vi "DeviceConfigType_to_Byte.vi"(4 "DeviceConfig":T1) -> (1 "Byte Array":u8[](array[numeric]))   [LabVIEW 2020]
uses:
  <instrlib>/Devices/Avantes/clusterdef.ctl
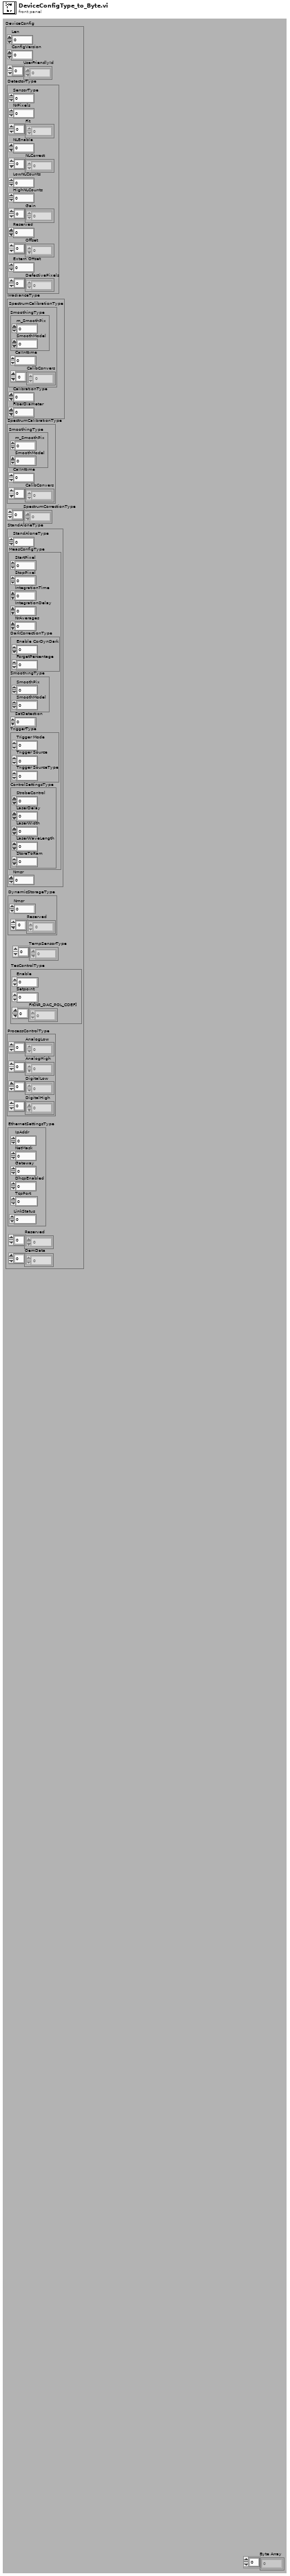
[diagram p1: front panel]
types:
  T1 = typedef "clusterdef.ctl" = cluster{"Len":u16, "ConfigVersion":u16, "UserFriendlyId":u8[], "DetectorType":cluster{"SensorType":u8, "NrPixels":u16, "Fit":sgl[], "NLEnable":u8, "NLCorrect":dbl[], "LowNLCounts":dbl, "HighNLCounts":dbl, "Gain":sgl[], "Reserved":sgl, "Offset":sgl[], "Extern Offset":sgl, "DefectivePixels":u16[]}, "IrradianceType":cluster{"SpectrumCalibrationType":cluster{"SmoothingType":cluster{"m_SmoothPix":u16, "SmoothModel":u8}, "CalInttime":sgl, "CalibConvers":sgl[]}, "CalibrationType":u8, "FiberDiameter":i32}, "SpectrumCalibrationType":cluster{"SmoothingType":cluster{"m_SmoothPix":u16, "SmoothModel":u8}, "CalInttime":sgl, "CalibConvers":sgl[]}, "SpectrumCorrectionType":sgl[], "StandAloneType":cluster{"StandAloneType":u8, "MeasConfigType":cluster{"StartPixel":u16, "StopPixel":u16, "IntegrationTime":sgl, "IntegrationDelay":u32, "NrAverages":u32, "DarkCorrectionType":cluster{"Enable CorDynDark":u8, "ForgetPercentage":u8}, "SmoothingType":cluster{"SmoothPix":u16, "SmoothModel":u8}, "SatDetection":u8, "TriggerType":cluster{"Trigger Mode":u8, "Trigger Source":u8, "Trigger SourceType":u8}, "ControlSettingsType":cluster{"StrobeControl":u16, "LaserDelay":u32, "LaserWidth":u32, "LaserWaveLength":sgl, "StoreToRam":u16}}, "Nmsr":i16}, "DynamicStorageType":cluster{"Nmsr":i32, "Reserved":u8[]}, "TempSensorType":sgl[], "TecControlType":cluster{"Enable":u8, "Setpoint":sgl, "Fit[NR_DAC_POL_COEF]":sgl[]}, "ProcessControlType":cluster{"AnalogLow":sgl[], "AnalogHigh":sgl[], "DigitalLow":sgl[], "DigitalHigh":sgl[]}, "EthernetSettingsType":cluster{"IpAddr":u32, "NetMask":u32, "Gateway":u32, "DhcpEnabled":u8, "TcpPort":u16, "LinkStatus":u8}, "Reserved":u8[], "OemData":u8[]}
  T2 = cluster{"SensorType":u8, "NrPixels":u16, "Fit":sgl[], "NLEnable":u8, "NLCorrect":dbl[], "LowNLCounts":dbl, "HighNLCounts":dbl, "Gain":sgl[], "Reserved":sgl, "Offset":sgl[], "Extern Offset":sgl, "DefectivePixels":u16[]}
  T3 = cluster{"SpectrumCalibrationType":cluster{"SmoothingType":cluster{"m_SmoothPix":u16, "SmoothModel":u8}, "CalInttime":sgl, "CalibConvers":sgl[]}, "CalibrationType":u8, "FiberDiameter":i32}
  T4 = cluster{"SmoothingType":cluster{"m_SmoothPix":u16, "SmoothModel":u8}, "CalInttime":sgl, "CalibConvers":sgl[]}
  T5 = cluster{"StandAloneType":u8, "MeasConfigType":cluster{"StartPixel":u16, "StopPixel":u16, "IntegrationTime":sgl, "IntegrationDelay":u32, "NrAverages":u32, "DarkCorrectionType":cluster{"Enable CorDynDark":u8, "ForgetPercentage":u8}, "SmoothingType":cluster{"SmoothPix":u16, "SmoothModel":u8}, "SatDetection":u8, "TriggerType":cluster{"Trigger Mode":u8, "Trigger Source":u8, "Trigger SourceType":u8}, "ControlSettingsType":cluster{"StrobeControl":u16, "LaserDelay":u32, "LaserWidth":u32, "LaserWaveLength":sgl, "StoreToRam":u16}}, "Nmsr":i16}
  T6 = cluster{"Enable":u8, "Setpoint":sgl, "Fit[NR_DAC_POL_COEF]":sgl[]}
  T7 = cluster{"AnalogLow":sgl[], "AnalogHigh":sgl[], "DigitalLow":sgl[], "DigitalHigh":sgl[]}
  T8 = cluster{"IpAddr":u32, "NetMask":u32, "Gateway":u32, "DhcpEnabled":u8, "TcpPort":u16, "LinkStatus":u8}
  T9 = cluster{"StartPixel":u16, "StopPixel":u16, "IntegrationTime":sgl, "IntegrationDelay":u32, "NrAverages":u32, "DarkCorrectionType":cluster{"Enable CorDynDark":u8, "ForgetPercentage":u8}, "SmoothingType":cluster{"SmoothPix":u16, "SmoothModel":u8}, "SatDetection":u8, "TriggerType":cluster{"Trigger Mode":u8, "Trigger Source":u8, "Trigger SourceType":u8}, "ControlSettingsType":cluster{"StrobeControl":u16, "LaserDelay":u32, "LaserWidth":u32, "LaserWaveLength":sgl, "StoreToRam":u16}}
  T10 = cluster{"Enable CorDynDark":u8, "ForgetPercentage":u8}
  T11 = cluster{"Trigger Mode":u8, "Trigger Source":u8, "Trigger SourceType":u8}
  T12 = cluster{"StrobeControl":u16, "LaserDelay":u32, "LaserWidth":u32, "LaserWaveLength":sgl, "StoreToRam":u16}
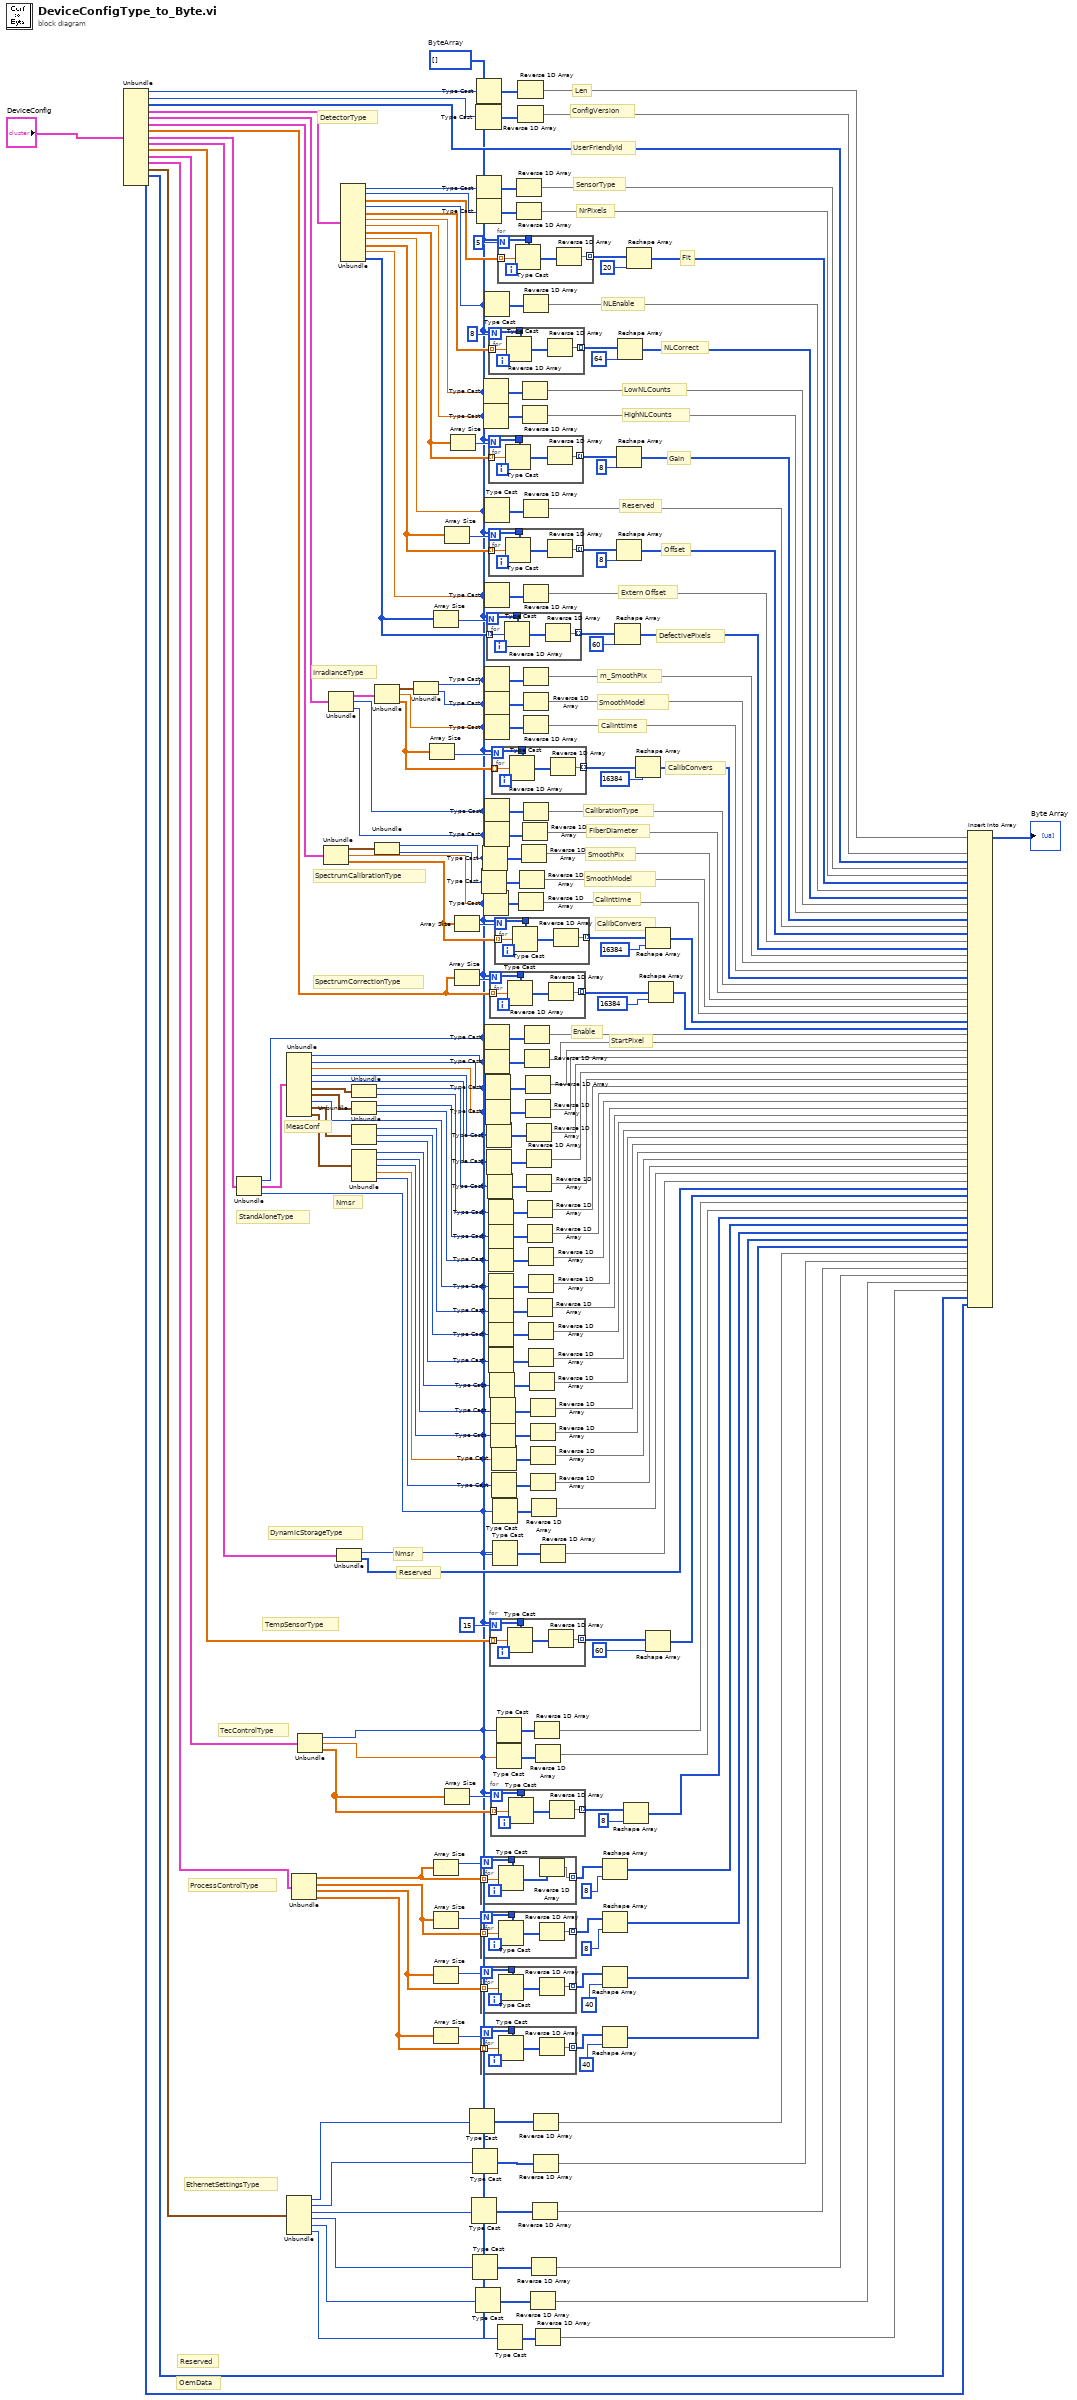
[diagram p0: block diagram]
diagram:
  w3 = u8[] []  # ByteArray
  # "OemData"
  # "Reserved"
  # "EthernetSettingsType"
  # "Reserved"
  # "Nmsr"
  # "DynamicStorageType"
  # "ProcessControlType"
  # "TecControlType"
  # "TempSensorType"
  # "Nmsr"
  # "MeasConf"
  # "StartPixel"
  # "Enable"
  # "StandAloneType"
  # "SpectrumCorrectionType"
  # "SpectrumCalibrationType"
  # "CalibConvers"
  # "CalInttime"
  # "SmoothModel"
  # "SmoothPix"
  # "FiberDiameter"
  # "CalibrationType"
  # "CalibConvers"
  # "CalInttime"
  # "SmoothModel"
  # "m_SmoothPix"
  # "IrradianceType"
  # "DefectivePixels"
  # "Extern Offset"
  # "Offset"
  # "Reserved"
  # "Gain"
  # "HighNLCounts"
  # "LowNLCounts"
  # "NLCorrect"
  # "NLEnable"
  # "Fit"
  # "NrPixels"
  # "SensorType"
  # "DetectorType"
  # "UserFriendlyId"
  # "ConfigVersion"
  # "Len"
  n1 = Unbundle("DeviceConfig") -> ("Len"=w226:u16, "ConfigVersion"=w225:u16, "UserFriendlyId"=w78:u8[], "DetectorType"=w224:T2, "IrradianceType"=w201:T3, "SpectrumCalibrationType"=w183:T4, "SpectrumCorrectionType"=w66:sgl[], "StandAloneType"=w174:T5, "DynamicStorageType"=w35:cluster{"Nmsr":i32, "Reserved":u8[]}, "TempSensorType"=w36:sgl[], "TecControlType"=w37:T6, "ProcessControlType"=w38:T7, "EthernetSettingsType"=w22:T8, "Reserved"=w2:u8[], "OemData"=w1:u8[])
  n2 = Unbundle(w174) -> ("StandAloneType"=w162:u8, "MeasConfigType"=w173:T9, "Nmsr"=w118:i16)
  n3 = Unbundle(w173) -> ("StartPixel"=w161:u16, "StopPixel"=w160:u16, "IntegrationTime"=w159:sgl, "IntegrationDelay"=w158:u32, "NrAverages"=w157:u32, "DarkCorrectionType"=w172:T10, "SmoothingType"=w171:cluster{"SmoothPix":u16, "SmoothModel":u8}, "SatDetection"=w147:u8, "TriggerType"=w170:T11, "ControlSettingsType"=w169:T12)
  n4 = Unbundle(w22) -> ("IpAddr"=w15:u32, "NetMask"=w14:u32, "Gateway"=w13:u32, "DhcpEnabled"=w18:u8, "TcpPort"=w17:u16, "LinkStatus"=w19:u8)
  n5 = Unbundle(w38) -> ("AnalogLow"=w52:sgl[], "AnalogHigh"=w48:sgl[], "DigitalLow"=w47:sgl[], "DigitalHigh"=w46:sgl[])
  n6 = Unbundle(w37) -> ("Enable"=w61:u8, "Setpoint"=w60:sgl, "Fit[NR_DAC_POL_COEF]"=w56:sgl[])
  n7 = Unbundle(w183) -> ("SmoothingType"=w182:cluster{"m_SmoothPix":u16, "SmoothModel":u8}, "CalInttime"=w177:sgl, "CalibConvers"=w65:sgl[])
  n8 = Unbundle(w201) -> ("SpectrumCalibrationType"=w200:T4, "CalibrationType"=w190:u8, "FiberDiameter"=w189:i32)
  n9 = Unbundle(w35) -> ("Nmsr"=w34:i32, "Reserved"=w31:u8[])
  n10 = Unbundle(w224) -> ("SensorType"=w221:u8, "NrPixels"=w223:u16, "Fit"=w76:sgl[], "NLEnable"=w216:u8, "NLCorrect"=w98:dbl[], "LowNLCounts"=w212:dbl, "HighNLCounts"=w211:dbl, "Gain"=w75:sgl[], "Reserved"=w210:sgl, "Offset"=w72:sgl[], "Extern Offset"=w207:sgl, "DefectivePixels"=w70:u16[])
  n11 = Unbundle(w172) -> ("Enable CorDynDark"=w151:u8, "ForgetPercentage"=w150:u8)
  n12 = Unbundle(w171) -> ("SmoothPix"=w149:u16, "SmoothModel"=w148:u8)
  n13 = Unbundle(w170) -> ("Trigger Mode"=w127:u8, "Trigger Source"=w126:u8, "Trigger SourceType"=w125:u8)
  n14 = Unbundle(w169) -> ("StrobeControl"=w124:u16, "LaserDelay"=w123:u32, "LaserWidth"=w122:u32, "LaserWaveLength"=w121:sgl, "StoreToRam"=w120:u16)
  n15 = Unbundle(w200) -> ("SmoothingType"=w199:cluster{"m_SmoothPix":u16, "SmoothModel":u8}, "CalInttime"=w191:sgl, "CalibConvers"=w68:sgl[])
  n16 = Unbundle(w182) -> ("m_SmoothPix"=w181:u16, "SmoothModel"=w178:u8)
  n17 = Unbundle(w199) -> ("m_SmoothPix"=w193:u16, "SmoothModel"=w192:u8)
  n18 = Array Size(array=w68) -> (size(s)=w69:i32)
  n19 = Array Size(array=w70) -> (size(s)=w71:i32)
  n20 = Array Size(array=w52) -> (size(s)=w55:i32)
  n21 = Array Size(array=w48) -> (size(s)=w49:i32)
  n22 = Array Size(array=w47) -> (size(s)=w50:i32)
  n23 = Array Size(array=w46) -> (size(s)=w51:i32)
  n24 = Array Size(array=w72) -> (size(s)=w73:i32)
  n25 = Array Size(array=w56) -> (size(s)=w57:i32)
  n26 = Array Size(array=w75) -> (size(s)=w74:i32)
  n27 = Array Size(array=w65) -> (size(s)=w64:i32)
  n28 = Array Size(array=w66) -> (size(s)=w67:i32)
  n29 = Type Cast(type=w3, x=w15) -> (*(type *) &x=w12:u8[])
  n30 = Type Cast(type=w3, x=w13) -> (*(type *) &x=w10:u8[])
  n31 = Type Cast(type=w3, x=w14) -> (*(type *) &x=w11:u8[])
  n32 = Type Cast(type=w3, x=w18) -> (*(type *) &x=w21:u8[])
  n33 = Type Cast(type=w3, x=w17) -> (*(type *) &x=w16:u8[])
  n34 = Type Cast(type=w3, x=w225) -> (*(type *) &x=w230:u8[])
  n35 = Type Cast(type=w3, x=w226) -> (*(type *) &x=w231:u8[])
  n36 = Type Cast(type=w3, x=w221) -> (*(type *) &x=w222:u8[])
  n37 = Type Cast(type=w3, x=w223) -> (*(type *) &x=w227:u8[])
  n38 = for {
    N: w55 -> [_]
    tunnel: w52 -> [w235] mode=indexing
    tunnel: [w234] -> w53 mode=indexing
    tunnel: w3 -> [w232]
    n39 = Type Cast(type=w232, x=w235) -> (*(type *) &x=w233:u8[])
    n40 = Reverse 1D Array(array=w233) -> (reversed array=w234:u8[])
  }
  n41 = for {
    N: w49 -> [_]
    tunnel: w48 -> [w239] mode=indexing
    tunnel: [w238] -> w45 mode=indexing
    tunnel: w3 -> [w236]
    n42 = Type Cast(type=w236, x=w239) -> (*(type *) &x=w237:u8[])
    n43 = Reverse 1D Array(array=w237) -> (reversed array=w238:u8[])
  }
  n44 = for {
    N: w50 -> [_]
    tunnel: w47 -> [w243] mode=indexing
    tunnel: [w242] -> w44 mode=indexing
    tunnel: w3 -> [w240]
    n45 = Type Cast(type=w240, x=w243) -> (*(type *) &x=w241:u8[])
    n46 = Reverse 1D Array(array=w241) -> (reversed array=w242:u8[])
  }
  n47 = for {
    N: w51 -> [_]
    tunnel: w46 -> [w247] mode=indexing
    tunnel: [w246] -> w43 mode=indexing
    tunnel: w3 -> [w244]
    n48 = Type Cast(type=w244, x=w247) -> (*(type *) &x=w245:u8[])
    n49 = Reverse 1D Array(array=w245) -> (reversed array=w246:u8[])
  }
  n50 = Type Cast(type=w3, x=w178) -> (*(type *) &x=w180:u8[])
  n51 = Type Cast(type=w3, x=w181) -> (*(type *) &x=w197:u8[])
  n52 = Type Cast(type=w3, x=w212) -> (*(type *) &x=w214:u8[])
  n53 = Type Cast(type=w3, x=w211) -> (*(type *) &x=w213:u8[])
  n54 = Type Cast(type=w3, x=w177) -> (*(type *) &x=w179:u8[])
  n55 = Type Cast(type=w3, x=w216) -> (*(type *) &x=w218:u8[])
  n56 = Type Cast(type=w3, x=w207) -> (*(type *) &x=w208:u8[])
  n57 = Type Cast(type=w3, x=w193) -> (*(type *) &x=w209:u8[])
  n58 = Type Cast(type=w3, x=w192) -> (*(type *) &x=w195:u8[])
  n59 = Type Cast(type=w3, x=w191) -> (*(type *) &x=w194:u8[])
  n60 = Type Cast(type=w3, x=w189) -> (*(type *) &x=w196:u8[])
  n61 = Type Cast(type=w3, x=w210) -> (*(type *) &x=w215:u8[])
  n62 = Type Cast(type=w3, x=w190) -> (*(type *) &x=w198:u8[])
  n63 = Type Cast(type=w3, x=w162) -> (*(type *) &x=w164:u8[])
  n64 = Type Cast(type=w3, x=w161) -> (*(type *) &x=w163:u8[])
  n65 = Type Cast(type=w3, x=w160) -> (*(type *) &x=w165:u8[])
  n66 = Type Cast(type=w3, x=w159) -> (*(type *) &x=w166:u8[])
  n67 = for {
    N: w71 -> [_]
    tunnel: w70 -> [w251] mode=indexing
    tunnel: [w250] -> w91 mode=indexing
    tunnel: w3 -> [w248]
    n68 = Type Cast(type=w248, x=w251) -> (*(type *) &x=w249:u8[])
    n69 = Reverse 1D Array(array=w249) -> (reversed array=w250:u8[])
  }
  n70 = Type Cast(type=w3, x=w158) -> (*(type *) &x=w167:u8[])
  n71 = Type Cast(type=w3, x=w157) -> (*(type *) &x=w168:u8[])
  n72 = Type Cast(type=w3, x=w151) -> (*(type *) &x=w156:u8[])
  n73 = for {
    N: w74 -> [_]
    tunnel: w75 -> [w255] mode=indexing
    tunnel: [w254] -> w97 mode=indexing
    tunnel: w3 -> [w252]
    n74 = Type Cast(type=w252, x=w255) -> (*(type *) &x=w253:u8[])
    n75 = Reverse 1D Array(array=w253) -> (reversed array=w254:u8[])
  }
  n76 = for {
    N: w73 -> [_]
    tunnel: w72 -> [w259] mode=indexing
    tunnel: [w258] -> w94 mode=indexing
    tunnel: w3 -> [w256]
    n77 = Type Cast(type=w256, x=w259) -> (*(type *) &x=w257:u8[])
    n78 = Reverse 1D Array(array=w257) -> (reversed array=w258:u8[])
  }
  n79 = Type Cast(type=w3, x=w150) -> (*(type *) &x=w155:u8[])
  n80 = Type Cast(type=w3, x=w149) -> (*(type *) &x=w154:u8[])
  n81 = Type Cast(type=w3, x=w127) -> (*(type *) &x=w130:u8[])
  n82 = for {
    N: 8 -> [_]
    tunnel: w98 -> [w263] mode=indexing
    tunnel: [w262] -> w101 mode=indexing
    tunnel: w3 -> [w260]
    n83 = Type Cast(type=w260, x=w263) -> (*(type *) &x=w261:u8[])
    n84 = Reverse 1D Array(array=w261) -> (reversed array=w262:u8[])
  }
  n85 = Type Cast(type=w3, x=w148) -> (*(type *) &x=w153:u8[])
  n86 = Type Cast(type=w3, x=w147) -> (*(type *) &x=w152:u8[])
  n87 = Type Cast(type=w3, x=w126) -> (*(type *) &x=w129:u8[])
  n88 = Type Cast(type=w3, x=w125) -> (*(type *) &x=w128:u8[])
  n89 = for {
    N: w67 -> [_]
    tunnel: w66 -> [w267] mode=indexing
    tunnel: [w266] -> w82 mode=indexing
    tunnel: w3 -> [w264]
    n90 = Type Cast(type=w264, x=w267) -> (*(type *) &x=w265:u8[])
    n91 = Reverse 1D Array(array=w265) -> (reversed array=w266:u8[])
  }
  n92 = Type Cast(type=w3, x=w124) -> (*(type *) &x=w131:u8[])
  n93 = for {
    N: 15 -> [_]
    tunnel: w36 -> [w268] mode=indexing
    tunnel: [w271] -> w104 mode=indexing
    tunnel: w3 -> [w269]
    n94 = Type Cast(type=w269, x=w268) -> (*(type *) &x=w270:u8[])
    n95 = Reverse 1D Array(array=w270) -> (reversed array=w271:u8[])
  }
  n96 = Type Cast(type=w3, x=w123) -> (*(type *) &x=w132:u8[])
  n97 = Type Cast(type=w3, x=w122) -> (*(type *) &x=w133:u8[])
  n98 = for {
    N: w57 -> [_]
    tunnel: w56 -> [w275] mode=indexing
    tunnel: [w274] -> w59 mode=indexing
    tunnel: w3 -> [w272]
    n99 = Type Cast(type=w272, x=w275) -> (*(type *) &x=w273:u8[])
    n100 = Reverse 1D Array(array=w273) -> (reversed array=w274:u8[])
  }
  n101 = for {
    N: w69 -> [_]
    tunnel: w68 -> [w279] mode=indexing
    tunnel: [w278] -> w88 mode=indexing
    tunnel: w3 -> [w276]
    n102 = Type Cast(type=w276, x=w279) -> (*(type *) &x=w277:u8[])
    n103 = Reverse 1D Array(array=w277) -> (reversed array=w278:u8[])
  }
  n104 = Type Cast(type=w3, x=w121) -> (*(type *) &x=w134:u8[])
  n105 = Type Cast(type=w3, x=w120) -> (*(type *) &x=w135:u8[])
  n106 = Type Cast(type=w3, x=w118) -> (*(type *) &x=w119:u8[])
  n107 = Type Cast(type=w3, x=w34) -> (*(type *) &x=w33:u8[])
  n108 = for {
    N: w64 -> [_]
    tunnel: w65 -> [w283] mode=indexing
    tunnel: [w282] -> w85 mode=indexing
    tunnel: w3 -> [w280]
    n109 = Type Cast(type=w280, x=w283) -> (*(type *) &x=w281:u8[])
    n110 = Reverse 1D Array(array=w281) -> (reversed array=w282:u8[])
  }
  n111 = Type Cast(type=w3, x=w61) -> (*(type *) &x=w63:u8[])
  n112 = Type Cast(type=w3, x=w60) -> (*(type *) &x=w62:u8[])
  n113 = for {
    N: 5 -> [_]
    tunnel: w76 -> [w287] mode=indexing
    tunnel: [w286] -> w107 mode=indexing
    tunnel: w3 -> [w284]
    n114 = Type Cast(type=w284, x=w287) -> (*(type *) &x=w285:u8[])
    n115 = Reverse 1D Array(array=w285) -> (reversed array=w286:u8[])
  }
  n116 = Type Cast(type=w3, x=w19) -> (*(type *) &x=w20:u8[])
  n117 = Reverse 1D Array(array=w222) -> (reversed array=w220:u8[])
  n118 = Reverse 1D Array(array=w227) -> (reversed array=w219:u8[])
  n119 = Reverse 1D Array(array=w231) -> (reversed array=w229:u8[])
  n120 = Reverse 1D Array(array=w230) -> (reversed array=w228:u8[])
  n121 = Reverse 1D Array(array=w179) -> (reversed array=w175:u8[])
  n122 = Reverse 1D Array(array=w180) -> (reversed array=w176:u8[])
  n123 = Reverse 1D Array(array=w197) -> (reversed array=w184:u8[])
  n124 = Reverse 1D Array(array=w214) -> (reversed array=w206:u8[])
  n125 = Reverse 1D Array(array=w213) -> (reversed array=w205:u8[])
  n126 = Reverse 1D Array(array=w196) -> (reversed array=w185:u8[])
  n127 = Reverse 1D Array(array=w218) -> (reversed array=w217:u8[])
  n128 = Reverse 1D Array(array=w215) -> (reversed array=w204:u8[])
  n129 = Reverse 1D Array(array=w208) -> (reversed array=w203:u8[])
  n130 = Reverse 1D Array(array=w209) -> (reversed array=w202:u8[])
  n131 = Reverse 1D Array(array=w195) -> (reversed array=w188:u8[])
  n132 = Reverse 1D Array(array=w194) -> (reversed array=w187:u8[])
  n133 = Reverse 1D Array(array=w198) -> (reversed array=w186:u8[])
  n134 = Reverse 1D Array(array=w164) -> (reversed array=w146:u8[])
  n135 = Reverse 1D Array(array=w163) -> (reversed array=w145:u8[])
  n136 = Reverse 1D Array(array=w165) -> (reversed array=w144:u8[])
  n137 = Reverse 1D Array(array=w166) -> (reversed array=w143:u8[])
  n138 = Reverse 1D Array(array=w167) -> (reversed array=w142:u8[])
  n139 = Reverse 1D Array(array=w168) -> (reversed array=w141:u8[])
  n140 = Reverse 1D Array(array=w156) -> (reversed array=w140:u8[])
  n141 = Reverse 1D Array(array=w155) -> (reversed array=w139:u8[])
  n142 = Reverse 1D Array(array=w154) -> (reversed array=w138:u8[])
  n143 = Reverse 1D Array(array=w130) -> (reversed array=w117:u8[])
  n144 = Reverse 1D Array(array=w153) -> (reversed array=w137:u8[])
  n145 = Reverse 1D Array(array=w152) -> (reversed array=w136:u8[])
  n146 = Reverse 1D Array(array=w129) -> (reversed array=w116:u8[])
  n147 = Reverse 1D Array(array=w128) -> (reversed array=w115:u8[])
  n148 = Reverse 1D Array(array=w131) -> (reversed array=w114:u8[])
  n149 = Reverse 1D Array(array=w132) -> (reversed array=w113:u8[])
  n150 = Reverse 1D Array(array=w133) -> (reversed array=w112:u8[])
  n151 = Reverse 1D Array(array=w134) -> (reversed array=w111:u8[])
  n152 = Reverse 1D Array(array=w135) -> (reversed array=w110:u8[])
  n153 = Reverse 1D Array(array=w16) -> (reversed array=w5:u8[])
  n154 = Reverse 1D Array(array=w119) -> (reversed array=w109:u8[])
  n155 = Reverse 1D Array(array=w21) -> (reversed array=w6:u8[])
  n156 = Reverse 1D Array(array=w10) -> (reversed array=w7:u8[])
  n157 = Reverse 1D Array(array=w12) -> (reversed array=w9:u8[])
  n158 = Reverse 1D Array(array=w11) -> (reversed array=w8:u8[])
  n159 = Reverse 1D Array(array=w63) -> (reversed array=w29:u8[])
  n160 = Reverse 1D Array(array=w62) -> (reversed array=w28:u8[])
  n161 = Reverse 1D Array(array=w20) -> (reversed array=w4:u8[])
  n162 = Reverse 1D Array(array=w33) -> (reversed array=w32:u8[])
  n163 = Reshape Array(w53, 8 ("dimension size")) -> (w26:u8[])
  n164 = Reshape Array(w45, 8 ("dimension size")) -> (w25:u8[])
  n165 = Reshape Array(w44, 40 ("dimension size")) -> (w24:u8[])
  n166 = Reshape Array(w43, 40 ("dimension size")) -> (w23:u8[])
  n167 = Reshape Array(w91, 60 ("dimension size")) -> (w89:u8[])
  n168 = Reshape Array(w97, 8 ("dimension size")) -> (w95:u8[])
  n169 = Reshape Array(w94, 8 ("dimension size")) -> (w92:u8[])
  n170 = Reshape Array(w101, 64 ("dimension size")) -> (w99:u8[])
  n171 = Reshape Array(w59, 8 ("dimension size")) -> (w27:u8[])
  n172 = Reshape Array(w107, 20 ("dimension size")) -> (w77:u8[])
  n173 = Reshape Array(w88, 16384 ("dimension size")) -> (w86:u8[])
  n174 = Reshape Array(w85, 16384 ("dimension size")) -> (w83:u8[])
  n175 = Reshape Array(w104, 60 ("dimension size")) -> (w30:u8[])
  n176 = Reshape Array(w82, 16384 ("dimension size")) -> (w79:u8[])
  n177 = Insert Into Array(array=w229, new element #1=w228, new element #2=w78, new element #3=w220, new element #4=w219, new element #5=w77, new element #6=w217, new element #7=w99, new element #8=w206, new element #9=w205, new element #10=w95, new element #11=w204, new element #12=w92, new element #13=w203, new element #14=w89, new element #15=w202, new element #16=w188, new element #17=w187, new element #18=w86, new element #19=w186, new element #20=w185, new element #21=w184, new element #22=w176, new element #23=w175, new element #24=w83, new element #25=w79, new element #26=w146, new element #27=w145, new element #28=w144, new element #29=w143, new element #30=w142, new element #31=w141, new element #32=w140, new element #33=w139, new element #34=w138, new element #35=w137, new element #36=w136, new element #37=w117, new element #38=w116, new element #39=w115, new element #40=w114, new element #41=w113, new element #42=w112, new element #43=w111, new element #44=w110, new element #45=w109, new element #46=w32, new element #47=w31, new element #48=w30, new element #49=w29, new element #50=w28, new element #51=w27, new element #52=w26, new element #53=w25, new element #54=w24, new element #55=w23, new element #56=w9, new element #57=w8, new element #58=w7, new element #59=w6, new element #60=w5, new element #61=w4, new element #62=w2, new element #63=w1) -> (→"Byte Array":u8[])  [unwired: 1 in]
